vi "Read Session.vi"(8 "error in (no error)":errorcluster, 11 "Scope PXI in":refnum<class "Scope PXI.lvclass">) -> (0 "error out":errorcluster, 2 "session":refnum<k15>, 3 "Scope PXI out":refnum<class "Scope PXI.lvclass">)   [LabVIEW 2023, in "Scope.lvlib" / "Scope PXI.lvlib" / "Scope PXI.lvclass"]
uses:
  Scope PXI.lvclass
  Scope PXI CFG/Scope PXI CFG.lvclass
  Scope Base/Scope Base.lvclass/Scope Base.ctl
  Scope PXI CFG/Scope PXI CFG.lvclass/Scope PXI CFG.ctl
  Scope PXI.lvclass/Scope PXI.ctl
  Scope Base/Scope Base.lvclass
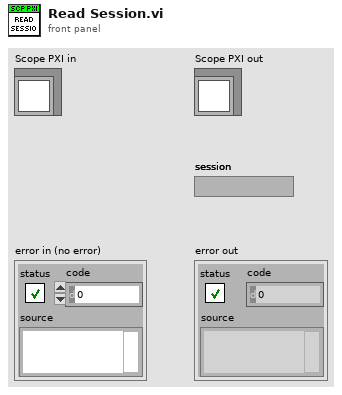
[diagram p1: front panel]
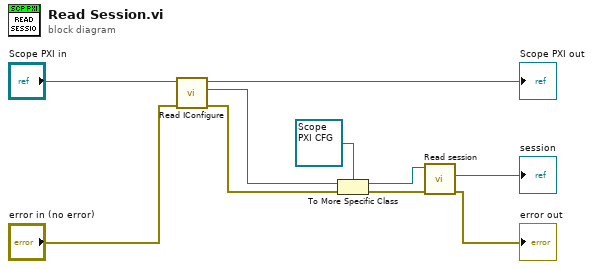
[diagram p0: block diagram]
diagram:
  n1 = call "Read IConfigure.vi"("error in (no error)"="error in (no error)", "Scope Base in"="Scope PXI in") -> ("error out"=w7:errorcluster, "IConfigureScope"=w5:refnum<class "IConfigure.lvclass">, "Scope Base out"=→"Scope PXI out":refnum<class "Scope PXI.lvclass">)  [unwired: 7 in]
  n2 = To More Specific Class(target class=refnum<class "Scope PXI CFG.lvclass"> refnum ("HAL.lvlib:Scope PXI CFG.lvclass"), reference=w5, error in=w7) -> (specific class reference=w3:refnum<class "Scope PXI CFG.lvclass">, error out=w6:errorcluster)
  n3 = call "Read session.vi"("error in (no error)"=w6, "Scope PXI CFG in"=w3) -> ("error out"=→"error out":errorcluster, "session"=→"session":refnum<k15>)  [unwired: 7 in, 1 out]
